vi "GObject Terminals.vi"(8 "error in (no error)":errorcluster, 11 "GObject in":refnum<vi>) -> (0 "error in (no error) (dup)":errorcluster, 1 "Class Name":string, 2 "Terms[]":refnum<vi>[](array[refnum]), 3 "Node Object":refnum<vi>, 4 "tunnel Relative Pos":T1)   [LabVIEW 2017, in "CSM-Helper.lvclass"]
uses:
  CSM-Helper.lvclass
  <vilib>/Utility/miscctls.llb/LVPositionTypeDef.ctl
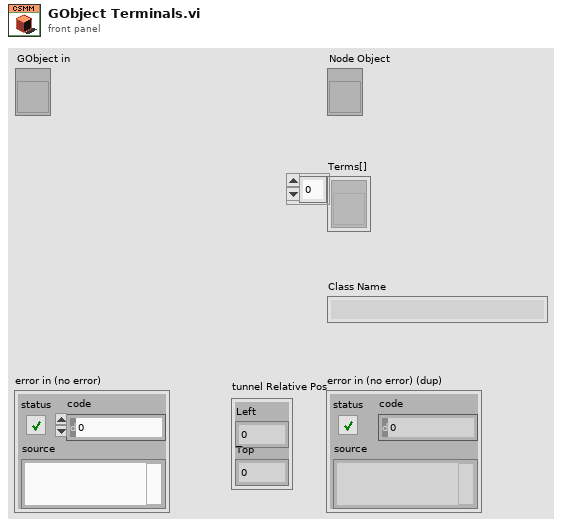
[diagram p1: front panel]
types:
  T1 = typedef "LVPositionTypeDef.ctl" = cluster{"Left":i32, "Top":i32}
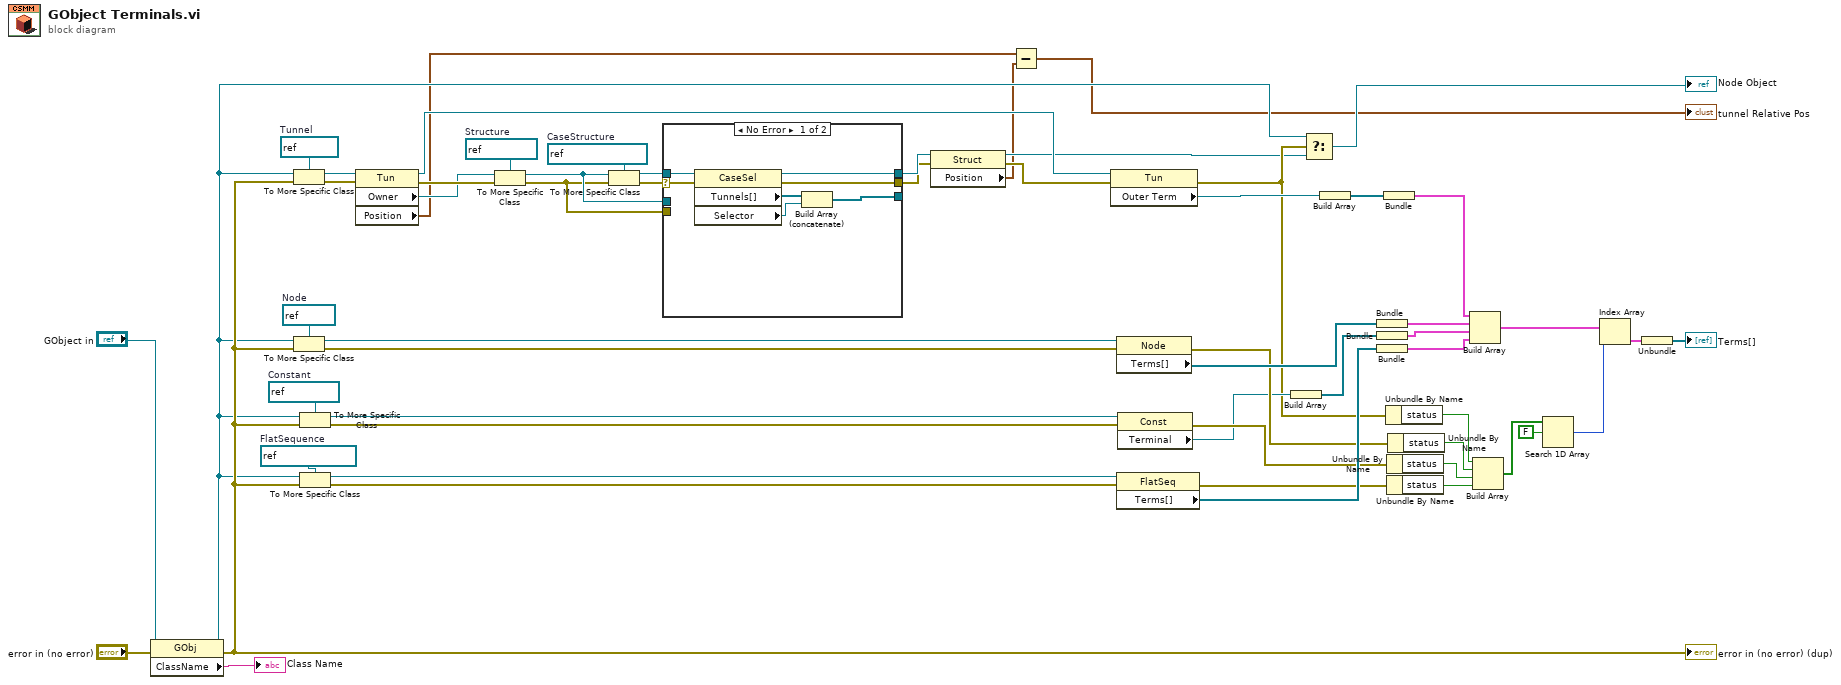
[diagram p0: block diagram]
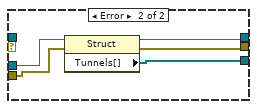
[diagram p2: hidden frame]
diagram:
  w11 = refnum<vi> refnum  # CaseStructure
  w17 = refnum<vi> refnum  # Structure
  w28 = refnum<vi> refnum  # Tunnel
  w41 = refnum<vi> refnum  # FlatSequence
  w38 = refnum<vi> refnum  # Constant
  w34 = refnum<vi> refnum  # Node
  n1 = property class="GObj"(reference="GObject in", error in="error in (no error)") -> (reference out=w13:refnum<vi>, error out=w22:errorcluster, "ClassName"=→"Class Name":string)
  "error in (no error) (dup)" <- w22
  n2 = To More Specific Class(target class=w28, reference=w13, error in=w22) -> (specific class reference=w21:refnum<vi>, error out=w20:errorcluster)
  n3 = To More Specific Class(target class=w34, reference=w13, error in=w22) -> (specific class reference=w33:refnum<vi>, error out=w32:errorcluster)
  n4 = To More Specific Class(target class=w38, reference=w13, error in=w22) -> (specific class reference=w36:refnum<vi>, error out=w35:errorcluster)
  n5 = To More Specific Class(target class=w41, reference=w13, error in=w22) -> (specific class reference=w42:refnum<vi>, error out=w43:errorcluster)
  n6 = property on="Property Node" class="Tun"(reference=w21, error in=w20) -> (reference out=w16:refnum<vi>, error out=w19:errorcluster, "Owner"=w18:refnum<vi>, "Position"=w3:T1)
  n7 = To More Specific Class(target class=w17, reference=w18, error in=w19) -> (specific class reference=w8:refnum<vi>, error out=w7:errorcluster)
  n8 = To More Specific Class(target class=w11, reference=w8, error in=w7) -> (specific class reference=w9:refnum<vi>, error out=w10:errorcluster)
  n9 = case shown="No Error" w10 {
    selector: w10 -> [w62 _]
    tunnel: [w65 w69] -> w5
    tunnel: [w60 w66] -> _
    tunnel: [w63 w67] -> w14
    tunnel: w9 -> [w61 _]
    tunnel: w8 -> [_ w70]
    tunnel: w7 -> [_ w68]
    frame No Error {
      n10 = property on="Property Node" class="CaseSel"(reference=w61, error in=w62) -> (reference out=w63:refnum<vi>, error out=w65:errorcluster, "Tunnels[]"=w64:refnum<vi>[], "Selector"=w59:refnum<vi>)
      n11 = Build Array (concatenate)(w64, w59) -> (w60:refnum<vi>[])
    }
    frame Error {
      n12 = property on="Property Node" class="Struct"(reference=w70, error in=w68) -> (reference out=w67:refnum<vi>, error out=w69:errorcluster, "Tunnels[]"=w66:refnum<vi>[])
    }
  }
  n13 = property class="Struct"(reference=w14, error in=w5) -> (reference out=w6:refnum<vi>, error out=w4:errorcluster, "Position"=w2:T1)
  n14 = Subtract(x=w3, y=w2) -> (x-y=→"tunnel Relative Pos":T1)
  n15 = property on="Property Node" class="Tun"(reference=w16, error in=w4) -> (error out=w15:errorcluster, "Outer Term"=w27:refnum<vi>)  [unwired: 1 out]
  n16 = property on="Property Node" class="Node"(reference=w33, error in=w32) -> (error out=w39:errorcluster, "Terms[]"=w50:refnum<vi>[])  [unwired: 1 out]
  n17 = property on="Property Node" class="FlatSeq"(reference=w42, error in=w43) -> (error out=w44:errorcluster, "Terms[]"=w52:refnum<vi>[])  [unwired: 1 out]
  n18 = property on="Property Node" class="Const"(reference=w36, error in=w35) -> (error out=w40:errorcluster, "Terminal"=w37:refnum<vi>)  [unwired: 1 out]
  n19 = Build Array(w37) -> (w51:refnum<vi>[])
  n20 = Select(t=w13, s=w15, f=w6) -> (s? t:f=→"Node Object":refnum<vi>)
  n21 = Build Array(w27) -> (w26:refnum<vi>[])
  n22 = Bundle("Terms[]"=w50) -> (w25:cluster{"Terms[]":refnum<vi>[]})  [unwired: 1 in]
  n23 = Bundle(w51) -> (w53:cluster{refnum<vi>[]})  [unwired: 1 in]
  n24 = Bundle("Terms[]"=w52) -> (w54:cluster{"Terms[]":refnum<vi>[]})  [unwired: 1 in]
  n25 = Bundle(w26) -> (w24:cluster{refnum<vi>[]})  [unwired: 1 in]
  n26 = Unbundle By Name(w15) -> ("status"=w23:bool)
  n27 = Unbundle By Name(w40) -> ("status"=w46:bool)
  n28 = Unbundle By Name(w44) -> ("status"=w47:bool)
  n29 = Unbundle By Name(w39) -> ("status"=w45:bool)
  n30 = Build Array(w24, w25, w53, w54) -> (w55:cluster{"Terms[]":refnum<vi>[]}[])
  n31 = Build Array(w23, w45, w46, w47) -> (w48:bool[])
  n32 = Search 1D Array(1D array=w48, element=FALSE) -> (index of element=w56:i32)  [unwired: 1 in]
  n33 = Index Array(array=w55, index=w56) -> (element=w57:cluster{"Terms[]":refnum<vi>[]})
  n34 = Unbundle(w57) -> ("Terms[]"=→"Terms[]":refnum<vi>[])
